vi "tcp_send.vi"(9 "Message JSON":string, 11 "Adresse du serveur":string) -> ()   [LabVIEW 2014]
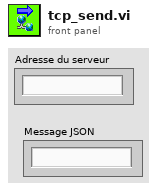
[diagram p1: front panel]
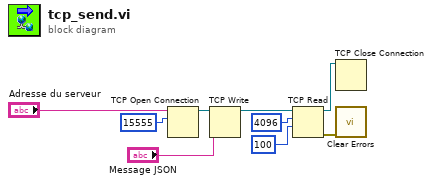
[diagram p0: block diagram]
diagram:
  n1 = TCP Open Connection(address="Adresse du serveur", remote port or service name=u16 15555) -> (connection ID=w4:refnum<k5>)  [unwired: 3 in, 1 out]
  n2 = TCP Write(connection ID=w4, data in="Message JSON") -> (connection ID out=w5:refnum<k5>)  [unwired: 2 in, 2 out]
  n3 = TCP Read(connection ID=w5, bytes to read=4096, 9:100 ("timeout ms (25000)")) -> (connection ID out=w7:refnum<k5>, error out=w9:errorcluster)  [unwired: 2 in, 1 out]
  n4 = TCP Close Connection(connection ID=w7) -> ()  [unwired: 2 in, 2 out]
  n5 = call <vilib>:"Clear Errors.vi"("error in (no error)"=w9) -> ()  [unwired: 5 in, 2 out]
